vi "compile_control_data_array.vi"(1 "dequeued data":T2={"Vapor Flow rate [g/s]"=0.0, "Liquid Flow rate [g/s]"=0.0, "Pressure/Temperature/Mixture Properties"={"Line Densities\n[g/cm^3]"={"Vapor Line"=-0.5709072724525495, "Liquid Line"=-0.47632842474153186}, "Mixture Properties"={"Enthalpy"=750619.9078232183, "Quality [-]"=0.5582470994443012}, "Component PTs"={"Liquid Tank P"=75343.41840909192, "Liquid Tank T"=30.52089213992321, "Liquid Tank Sat P"=181672.1439612281, "Liquid Tank Sat T"=6.822433775844459, "Separator P"=74401.45263172078, "Separator T"=37.19266445537589, "Separator Sat P"=233689.11712149414, "Separator Sat T"=6.478325372998782, "Liquid Inlet P"=82835.85841564724, "Liquid Inlet T"=193.56636718774698, "Liquid Inlet Sat P"=85427705.90320142, "Liquid Inlet Sat T"=9.415449685318322, "Vapor Tank P"=97469.18687679394, "Vapor Tank T"=6.224572479514193, "Vapor Tank Sat P"=72622.70102329315, "Vapor Tank Sat T"=13.864813139764351, "Vapor Inlet P"=182393.24586324493, "Vapor Inlet T"=24.91728208875432, "Vapor Inlet Sat P"=147043.33437190636, "Vapor Inlet Sat T"=31.003861452545706, "Test Section P"=nan, "Test Section T"=nan, "Test Section Sat P"=nan, "Test Section Sat T"=nan, "Upper Dev Section P"=14144.091653823736, "Upper Dev Section T"=549.9665015569866, "Upper Dev Section Sat P"=59290643216604.28, "Upper Dev Section Sat T"=-38.9295482785942, "Lower Dev Section P"=11233.297245789605, "Lower Dev Section T"=-2772.217721215085, "Lower Dev Section Sat P"=2.101296208665166e-41, "Lower Dev Section Sat T"=-45.23166544765655}, "Ambient Pressure [Pa]"=34261.54460917978, "Mixing Tee"={"Venturi dP"=0.0, "PGminiPressure"=0.0, "PGminiTemperature"=0.0}}, "Seconds Since \nSession Start"=0.0, "Raw Data Array"=[]}) -> (0 "control data array":dbl[](array[numeric]))   [LabVIEW 2017]
uses:
  pressure_temp_mixture.ctl
panel:
  # "Saturation\nPressure [Pa]"
  # "Saturation\nTemperature [C]"
  # "Pressure [Pa]"
  # "Temperature [C]"
  # "Liquid Tank"
  # "Separator"
  # "Liquid Inlet"
  # "Vapor Tank"
  # "Vapor Inlet"
  # "Test Section"
  # "Upper Dev Section"
  # "Lower Dev Section"
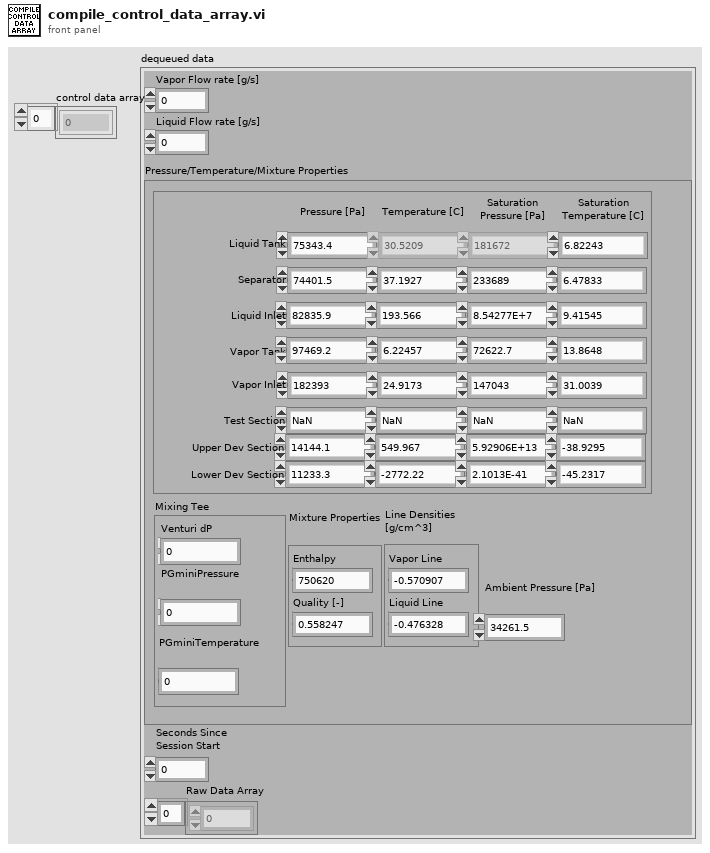
[diagram p1: front panel]
types:
  T1 = typedef "pressure_temp_mixture.ctl" = cluster{"Line Densities\n[g/cm^3]":cluster{"Vapor Line":dbl, "Liquid Line":dbl}, "Mixture Properties":cluster{"Enthalpy":dbl, "Quality [-]":dbl}, "Component PTs":cluster{"Liquid Tank P":dbl, "Liquid Tank T":dbl, "Liquid Tank Sat P":dbl, "Liquid Tank Sat T":dbl, "Separator P":dbl, "Separator T":dbl, "Separator Sat P":dbl, "Separator Sat T":dbl, "Liquid Inlet P":dbl, "Liquid Inlet T":dbl, "Liquid Inlet Sat P":dbl, "Liquid Inlet Sat T":dbl, "Vapor Tank P":dbl, "Vapor Tank T":dbl, "Vapor Tank Sat P":dbl, "Vapor Tank Sat T":dbl, "Vapor Inlet P":dbl, "Vapor Inlet T":dbl, "Vapor Inlet Sat P":dbl, "Vapor Inlet Sat T":dbl, "Test Section P":dbl, "Test Section T":dbl, "Test Section Sat P":dbl, "Test Section Sat T":dbl, "Upper Dev Section P":dbl, "Upper Dev Section T":dbl, "Upper Dev Section Sat P":dbl, "Upper Dev Section Sat T":dbl, "Lower Dev Section P":dbl, "Lower Dev Section T":dbl, "Lower Dev Section Sat P":dbl, "Lower Dev Section Sat T":dbl}, "Ambient Pressure [Pa]":dbl, "Mixing Tee":cluster{"Venturi dP":dbl, "PGminiPressure":dbl, "PGminiTemperature":dbl}}
  T2 = cluster{"Vapor Flow rate [g/s]":dbl, "Liquid Flow rate [g/s]":dbl, "Pressure/Temperature/Mixture Properties":T1, "Seconds Since \nSession Start":dbl, "Raw Data Array":dbl[]}
  T3 = cluster{"Liquid Tank P":dbl, "Liquid Tank T":dbl, "Liquid Tank Sat P":dbl, "Liquid Tank Sat T":dbl, "Separator P":dbl, "Separator T":dbl, "Separator Sat P":dbl, "Separator Sat T":dbl, "Liquid Inlet P":dbl, "Liquid Inlet T":dbl, "Liquid Inlet Sat P":dbl, "Liquid Inlet Sat T":dbl, "Vapor Tank P":dbl, "Vapor Tank T":dbl, "Vapor Tank Sat P":dbl, "Vapor Tank Sat T":dbl, "Vapor Inlet P":dbl, "Vapor Inlet T":dbl, "Vapor Inlet Sat P":dbl, "Vapor Inlet Sat T":dbl, "Test Section P":dbl, "Test Section T":dbl, "Test Section Sat P":dbl, "Test Section Sat T":dbl, "Upper Dev Section P":dbl, "Upper Dev Section T":dbl, "Upper Dev Section Sat P":dbl, "Upper Dev Section Sat T":dbl, "Lower Dev Section P":dbl, "Lower Dev Section T":dbl, "Lower Dev Section Sat P":dbl, "Lower Dev Section Sat T":dbl}
  T4 = cluster{"Venturi dP":dbl, "PGminiPressure":dbl, "PGminiTemperature":dbl}
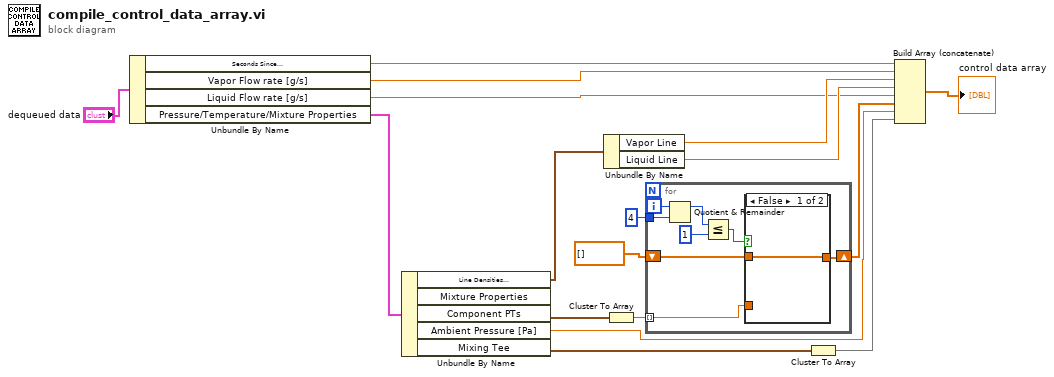
[diagram p0: block diagram]
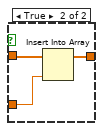
[diagram p2: hidden frame]
diagram:
  n1 = Unbundle By Name("dequeued data") -> ("Seconds Since \nSession Start"=w12:dbl, "Vapor Flow rate [g/s]"=w11:dbl, "Liquid Flow rate [g/s]"=w8:dbl, "Pressure/Temperature/Mixture Properties"=w16:T1)
  n2 = Unbundle By Name(w16) -> ("Line Densities\n[g/cm^3]"=w13:cluster{"Vapor Line":dbl, "Liquid Line":dbl}, "Component PTs"=w15:T3, "Ambient Pressure [Pa]"=w2:dbl, "Mixing Tee"=w14:T4)  [unwired: 1 out]
  n3 = Unbundle By Name(w13) -> ("Vapor Line"=w10:dbl, "Liquid Line"=w9:dbl)
  n4 = Cluster To Array(cluster=w15) -> (array=w7:dbl[])
  n5 = for {
    tunnel: w7 -> [w19] mode=indexing
    tunnel: 4 ("y") -> [w24]
    shift-right: [w18] -> w4
    shift-left: dbl[] [] -> [w20]
    i -> [w25]
    n6 = Quotient & Remainder(x=w25, y=w24) -> (x-y*floor(x/y)=w23:i32)  [unwired: 1 out]
    n7 = Less Or Equal?(x=w23, y=1) -> (x <= y?=w21:bool)
    n8 = case shown="False" w21 {
      tunnel: w20 -> [w26 w29]
      tunnel: w19 -> [_ w28]
      tunnel: [w26 w27] -> w18
      frame False {
      }
      frame True {
        n9 = Insert Into Array(array=w29, new element=w28) -> (w27:dbl[])  [unwired: 1 in]
      }
    }
  }
  n10 = Cluster To Array(cluster=w14) -> (array=w3:dbl[])
  n11 = Build Array (concatenate)(w12, w11, w10, w9, w8, w4, w2, w3) -> (→"control data array":dbl[])
